vi "VI Server_MenuRing_Update_ItemNames.vi"(7 "Label":string, 8 "error in":errorcluster, 10 "Strings []":string[](array[string]), 11 "VI Server Cluster":T1) -> (0 "error out":errorcluster, 1 "Control Reference":refnum<vi>, 3 "VI Server Cluster.DUP":T1)   [LabVIEW 2020, in "VI Server Toolkit LV2013.lvlib"]
doc: "Updates Menu Ring Items List."
uses:
  VI Server Toolkit LV2013.lvlib
  VI Server_TypeDefs/VI Server_RefsCluster.ctl
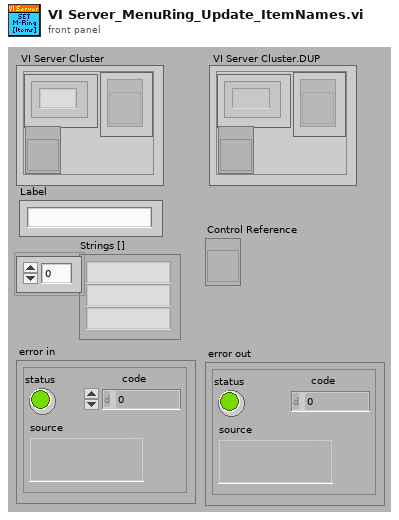
[diagram p1: front panel]
types:
  T1 = typedef "VI Server_RefsCluster.ctl" = cluster{"Labels":string[], "Refs":refnum<vi>[], "VI Ref":refnum<vi>}
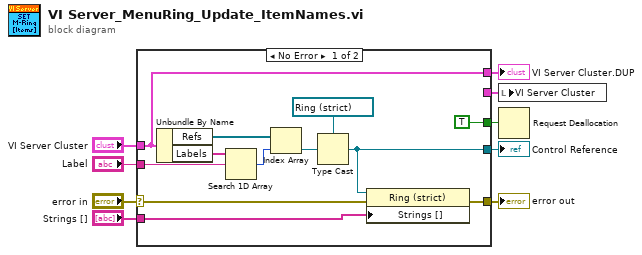
[diagram p0: block diagram]
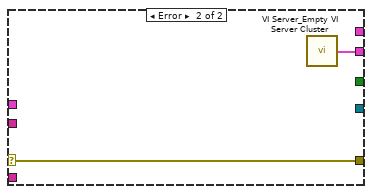
[diagram p2: hidden frame]
diagram:
  n1 = case shown="No Error" "error in" {
    selector: "error in" -> [w16 w23]
    tunnel: "Label" -> [w20 _]
    tunnel: "VI Server Cluster" -> [w11 _]
    tunnel: [w15 w23] -> w9
    tunnel: [w14 _] -> w5
    tunnel: "Strings []" -> [w13 _]
    tunnel: [w11 _] -> w3
    tunnel: [TRUE _] -> w2
    tunnel: [_ w22] -> w1
    frame No Error {
      n2 = Unbundle By Name(w11) -> ("Refs"=w18:refnum<vi>[], "Labels"=w21:string[])
      n3 = Search 1D Array(1D array=w21, element=w20) -> (index of element=w19:i32)  [unwired: 1 out]
      n4 = Index Array(array=w18, index=w19) -> (element=w17:refnum<vi>)
      n5 = Type Cast(type=refnum<vi> refnum ("Ring"), x=w17) -> (*(type *) &x=w14:refnum<vi>)
      n6 = property class="Ring (strict)"(reference=w14, error in=w16, "Strings []"=w13) -> (error out=w15:errorcluster)  [unwired: 1 out]
    }
    frame Error {
      n7 = call "VI Server_Empty VI Server Cluster.vi"() -> ("VI Server Cluster"=w22:T1)  [unwired: 7 in]
    }
  }
  "error out" <- w9
  "VI Server Cluster.DUP" <- w3
  "Control Reference" <- w5
  n8 = local write "VI Server Cluster"(w1) -> ()
  n9 = Request Deallocation(w2) -> ()
